vi "Transformer Turn Calculator.vi"() -> ()   [LabVIEW 2013]
panel:
  out "Turns Ratio":dbl
  in  "Power VA":dbl=50.0
  in  "Output Voltage":dbl=48.0
  in  "Input voltage":dbl=240.0
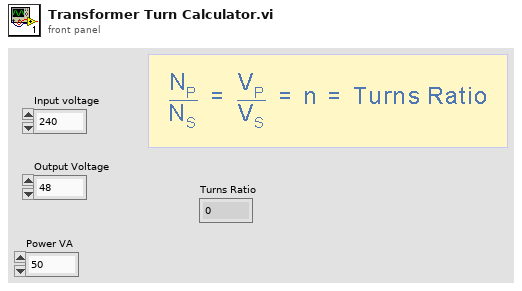
[diagram p1: front panel]
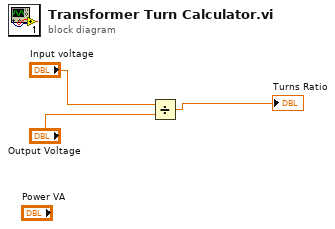
[diagram p0: block diagram]
diagram:
  n1 = Divide(x="Input voltage", y="Output Voltage") -> (x/y=→"Turns Ratio":dbl)
